vi "FTW-Crypto-PublicKeySignature-Verify.vi"(0 "Data":string="Data to encrypt!", 5 "Hex Encoded Signature":string, 7 "Public Key":string, 11 "error in":errorcluster) -> (4 "Signature Verified":bool, 15 "error out":errorcluster)   [LabVIEW 2015]
panel:
  # "Inputs"
  # "Outputs"
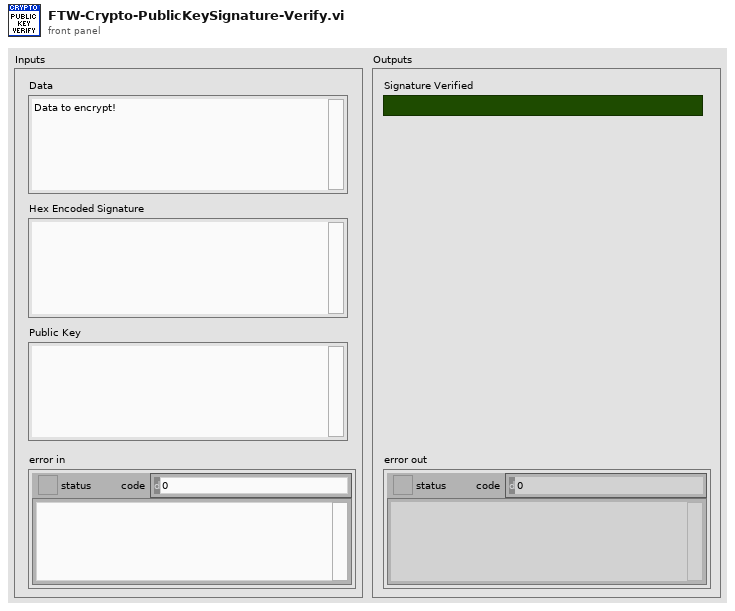
[diagram p1: front panel]
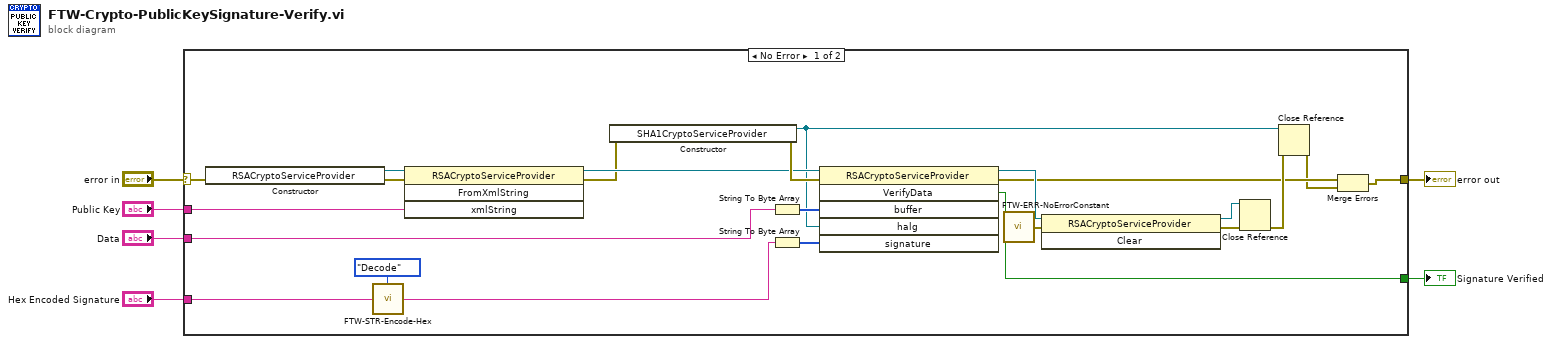
[diagram p0: block diagram]
diagram:
  n1 = case shown="No Error" "error in" {
    selector: "error in" -> [w29 w30]
    tunnel: "Data" -> [w28 _]
    tunnel: "Hex Encoded Signature" -> [w17 _]
    tunnel: [w8 w30] -> w3
    tunnel: [w25 _] -> w2
    tunnel: "Public Key" -> [w19 _]
    frame No Error {
      n2 = constructor class="RSACryptoServiceProvider"(error in=w29) -> (reference out=w23:refnum<k24>, error out=w21:errorcluster)  [unwired: 2 in, 1 out]
      n3 = call "FTW-STR-Encode-Hex.vi"("Input"=w17, "Direction"=enum16{"Encode", "Decode"}."Decode") -> ("Output"=w16:string)
      n4 = invoke class="RSACryptoServiceProvider" method="FromXmlString"(reference=w23, error in=w21, "xmlString"=w19) -> (reference out=w22:refnum<k24>, error out=w20:errorcluster)  [unwired: 1 in, 2 out]
      n5 = constructor class="SHA1CryptoServiceProvider"(error in=w20) -> (reference out=w12:refnum<k24>, error out=w26:errorcluster)  [unwired: 2 in, 1 out]
      n6 = String To Byte Array(string=w28) -> (unsigned byte array=w27:u8[])
      n7 = String To Byte Array(string=w16) -> (unsigned byte array=w24:u8[])
      n8 = invoke class="RSACryptoServiceProvider" method="VerifyData"(reference=w22, error in=w26, "buffer"=w27, "halg"=w12, "signature"=w24) -> (reference out=w15:refnum<k24>, error out=w10:errorcluster, "VerifyData"=w25:bool)  [unwired: 1 in, 3 out]
      n9 = call "FTW-ERR-NoErrorConstant.vi"() -> ("no error"=w7:errorcluster)
      n10 = invoke class="RSACryptoServiceProvider" method="Clear"(reference=w15, error in=w7) -> (reference out=w14:refnum<k24>, error out=w13:errorcluster)  [unwired: 1 in, 1 out]
      n11 = Close Reference(reference=w14, error in (no error)=w13) -> (error out=w11:errorcluster)
      n12 = Close Reference(reference=w12, error in (no error)=w11) -> (error out=w9:errorcluster)
      n13 = Merge Errors(w10, w9) -> (w8:errorcluster)
    }
    frame Error {
    }
  }
  "error out" <- w3
  "Signature Verified" <- w2
